vi "Execute.vi"(8 "error in (no error)":errorcluster, 9 "Consumer Queues in":T1, 10 "UI Process Command in":refnum<class "Generic UI Process Command.lvclass">, 11 "UI Process Data in":T2) -> (0 "error out":errorcluster, 1 "Consumer Queues out":T1, 2 "Stop?":bool, 3 "UI Process Data out":T2)   [LabVIEW 2019, in "User Interface Process.lvlib" / "Generic UI Process Command.lvclass"]
uses:
  Generic UI Process Command.lvclass
  UI Process Data.ctl
  TS Framework/ExeLogging/UI Logger/UI Logger.lvclass
  UI State.ctl
  TS Framework/Consumer Queues.ctl
  DAC Process/Generic DAC Command/Generic DAC Process Command.lvclass
  Trig Process/Generic Trig Command/Generic Trig Process Command.lvclass
  Generic UI Process Command.lvclass/Generic UI Process Command.ctl
  User Interface Process.lvlib
  TS Framework/TS Framework.lvlib
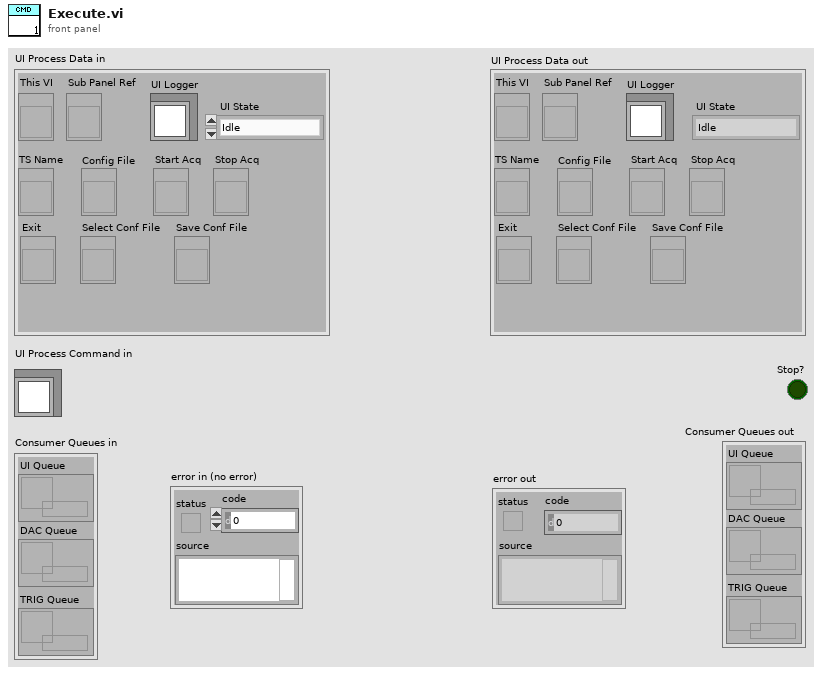
[diagram p1: front panel]
types:
  T1 = typedef "TS Framework.lvlib/Consumer Queues.ctl" = cluster{"UI Queue":refnum<queue>, "DAC Queue":refnum<queue>, "TRIG Queue":refnum<queue>}
  T2 = typedef "User Interface Process.lvlib/UI Process Data.ctl" = cluster{"This VI":refnum<vi>, "Sub Panel Ref":refnum<vi>, "UI Logger":refnum<class "UI Logger.lvclass">, "TS Name":refnum<vi>, "Config File":refnum<vi>, "Start Acq":refnum<vi>, "Stop Acq":refnum<vi>, "Exit":refnum<vi>, "Select Conf File":refnum<vi>, "Save Conf File":refnum<vi>, "UI State":T3}
  T3 = typedef "User Interface Process.lvlib/UI State.ctl" = enum16{"Idle", "Acquiring"}
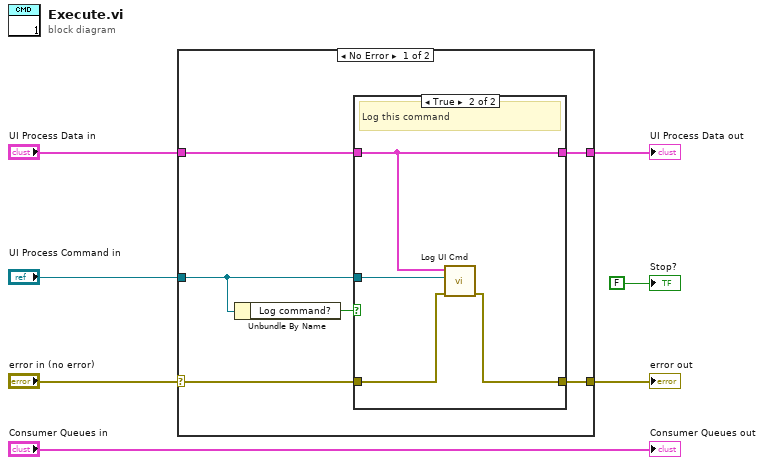
[diagram p0: block diagram]
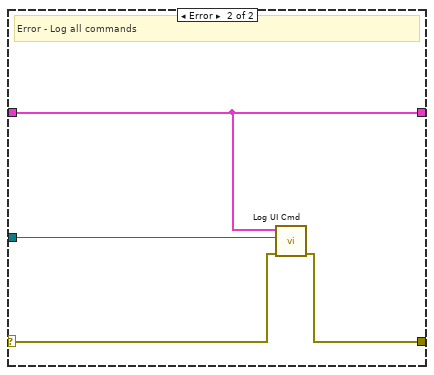
[diagram p3: hidden frame]
diagram:
  n1 = case shown="No Error" "error in (no error)" {
    selector: "error in (no error)" -> [w8 w22]
    tunnel: "UI Process Data in" -> [w13 w20]
    tunnel: [w12 w20] -> w4
    tunnel: [w11 w21] -> w3
    tunnel: "UI Process Command in" -> [w10 w23]
    frame No Error {
      n2 = Unbundle By Name(w10) -> ("Log command?"=w9:bool)
      n3 = case shown="True" w9 {
        tunnel: w13 -> [w15 w18]
        tunnel: [w15 w18] -> w12
        tunnel: w8 -> [w14 w17]
        tunnel: [w14 w16] -> w11
        tunnel: w10 -> [_ w19]
        frame False {
          # "Don't log this command"
        }
        frame True {
          # "Log this command"
          n4 = call "Log UI Cmd.vi"("error in (no error)"=w17, "UI Process Command in"=w19, "UI Process Data in"=w18) -> ("error out"=w16:errorcluster)  [unwired: 7 in, 1 out]
        }
      }
    }
    frame Error {
      # "Error - Log all commands"
      n5 = call "Log UI Cmd.vi"("error in (no error)"=w22, "UI Process Command in"=w23, "UI Process Data in"=w20) -> ("error out"=w21:errorcluster)  [unwired: 7 in, 1 out]
    }
  }
  "error out" <- w3
  "UI Process Data out" <- w4
  "Stop?" <- FALSE
  "Consumer Queues out" <- "Consumer Queues in"
